vi "Hf Generator - Copy.vi"(4 "Upper Frequency":dbl, 5 "Mic B Comp Fact":dbl, 6 "Speaker Device":dbl, 7 "Mic B":u32, 8 "Duration":dbl) -> (0 "Done":bool, 1 "Outlier Indexes":i32[](array[numeric]), 2 "df":dbl format="%0.2f", 3 "H(f)":cdb[](array[numeric]))   [LabVIEW 2018, in "Impedance Tube.lvlib"]
uses:
  Impedance Tube.lvlib
  <vilib>/sound2/lvsound2.llb/Sound Data Format.ctl
  <vilib>/sound2/lvsound2.llb/Sampling Mode.ctl
  <vilib>/Analysis/4window.llb/windowTd.ctl
  <vilib>/Analysis/6fits.llb/Remove Outliers (Range).vi
  <vilib>/sound2/lvsound2.llb/Sound Input Read (DBL).vi
  <vilib>/measure/maspectr.llb/Frequency Response Function (Real-Im) 1-1.vi
  <vilib>/Analysis/NI_AALPro.lvlib
  <vilib>/measure/NI_MAPro.lvlib
panel:
  out "Waveform Graph 2":dynamicdata(graph)
  out "Waveform Graph":dynamicdata(graph)
  out "Fi":dbl[](graph)
  out "Coherence":cluster{"f0":dbl, "df":dbl, "coherence":dbl[]}(graph)
  out "Numeric":dbl
  out "Frequency  2":cluster{dbl, dbl, dbl[]}(graph)
  out "averages completed":dbl format="%.2p"
  out "initialized array":dbl[](array[numeric])
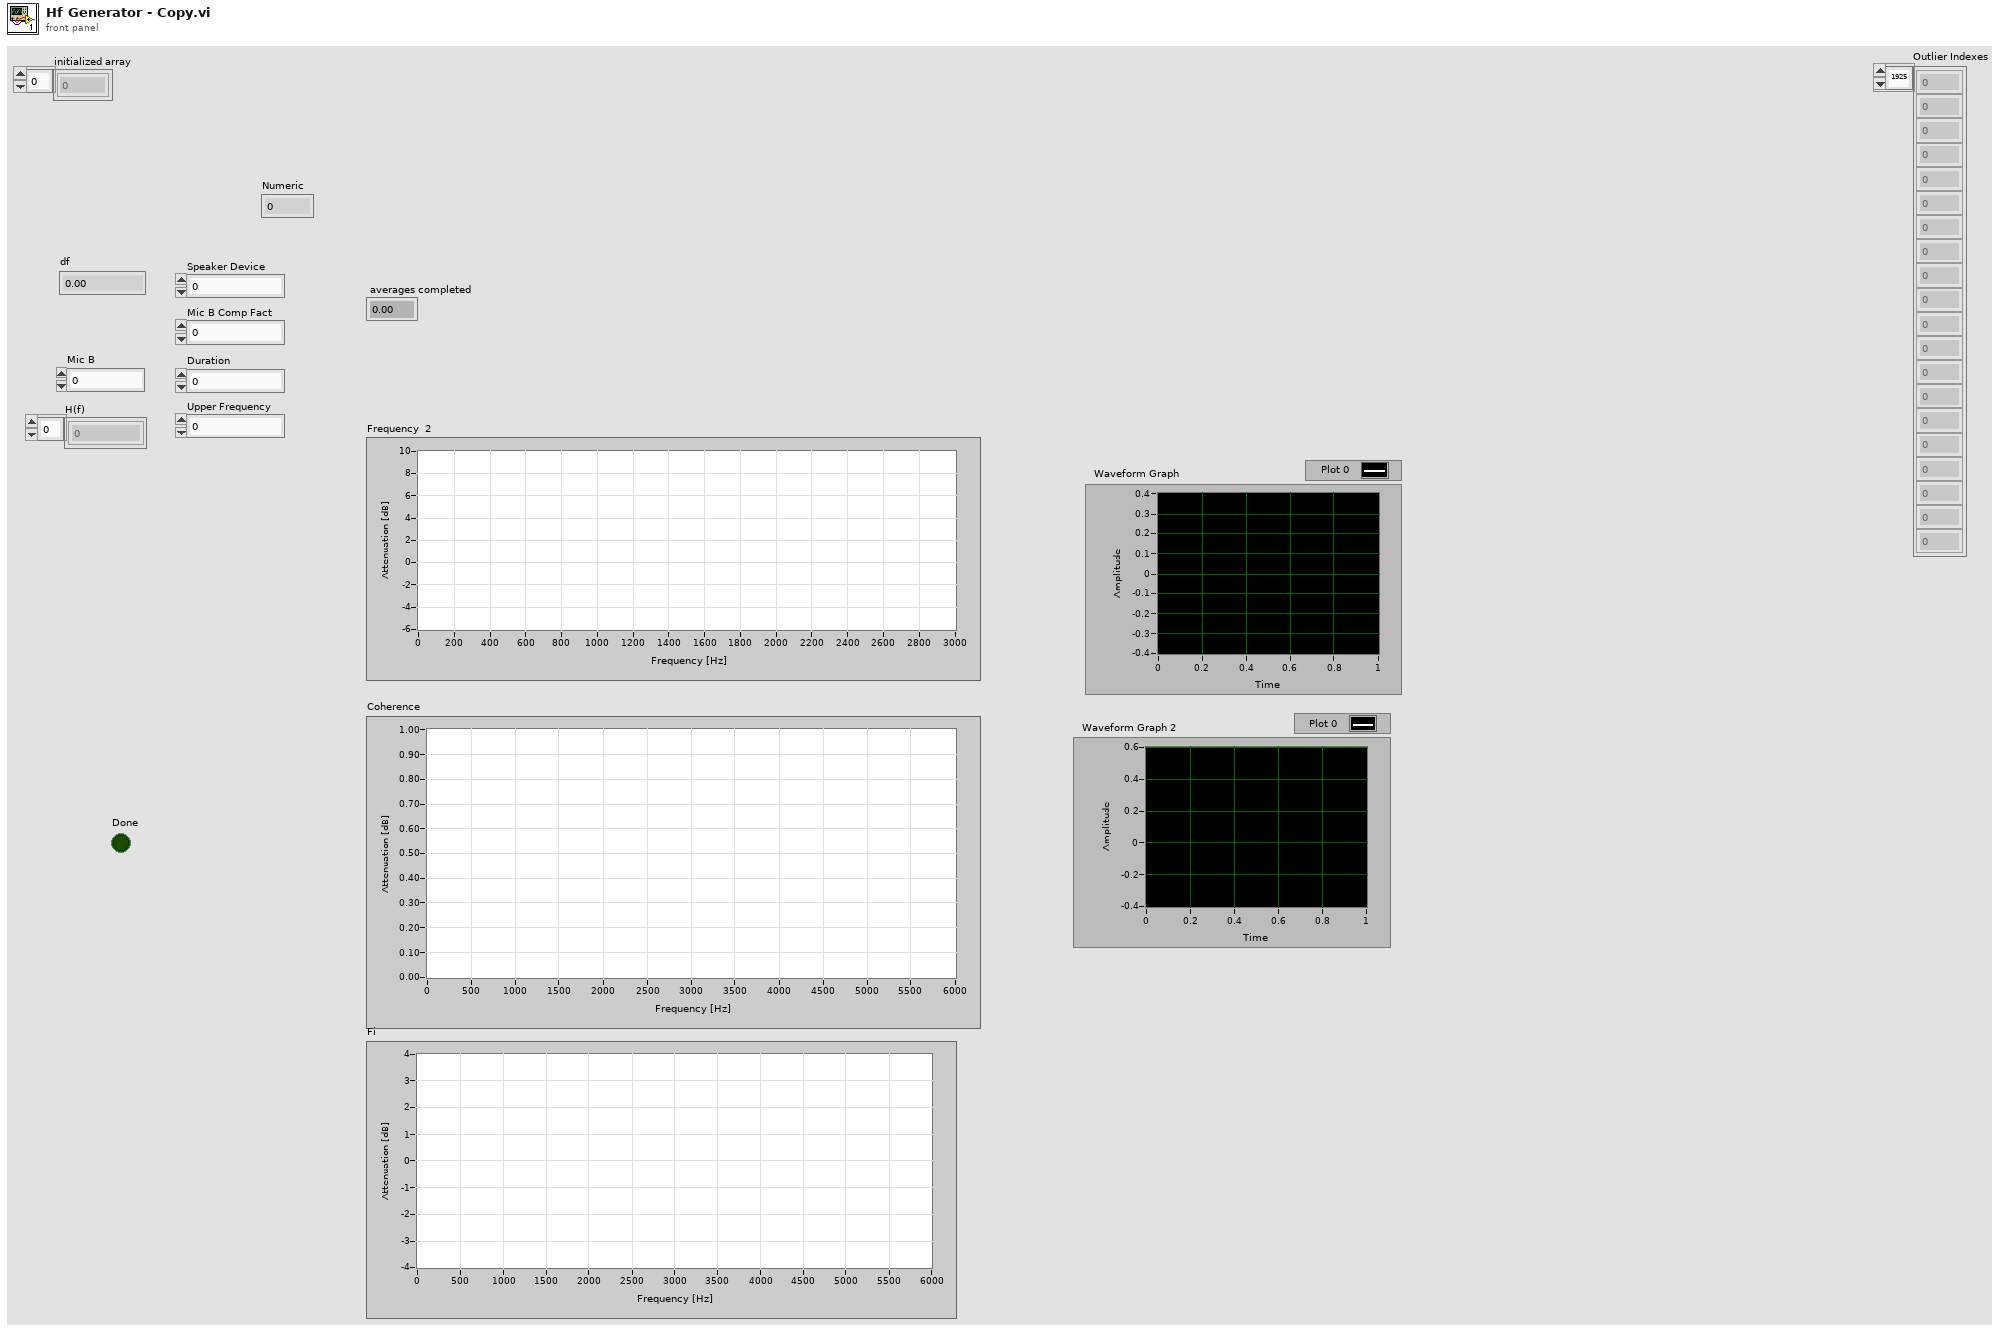
[diagram p1: front panel]
types:
  T1 = cluster{"averaging mode":enum16{"No averaging", "Vector averaging", "RMS averaging", "Peak hold"}, "weighting mode":enum16{"Linear", "Exponential"}, "number of averages":u32}
  T2 = typedef "Sampling Mode.ctl" = i32
  T3 = typedef "Sound Data Format.ctl" = cluster{"sample rate (S/s)":dbl, "number of channels":i32, "bits per sample":i32}
  T4 = typedef "Sound Input Task ID.ctl" = u32
  T5 = typedef "NI_AALPro.lvlib/windowTd.ctl" = u32
  T6 = cluster{"f0":dbl, "df":dbl, "imaginary part":dbl[]}
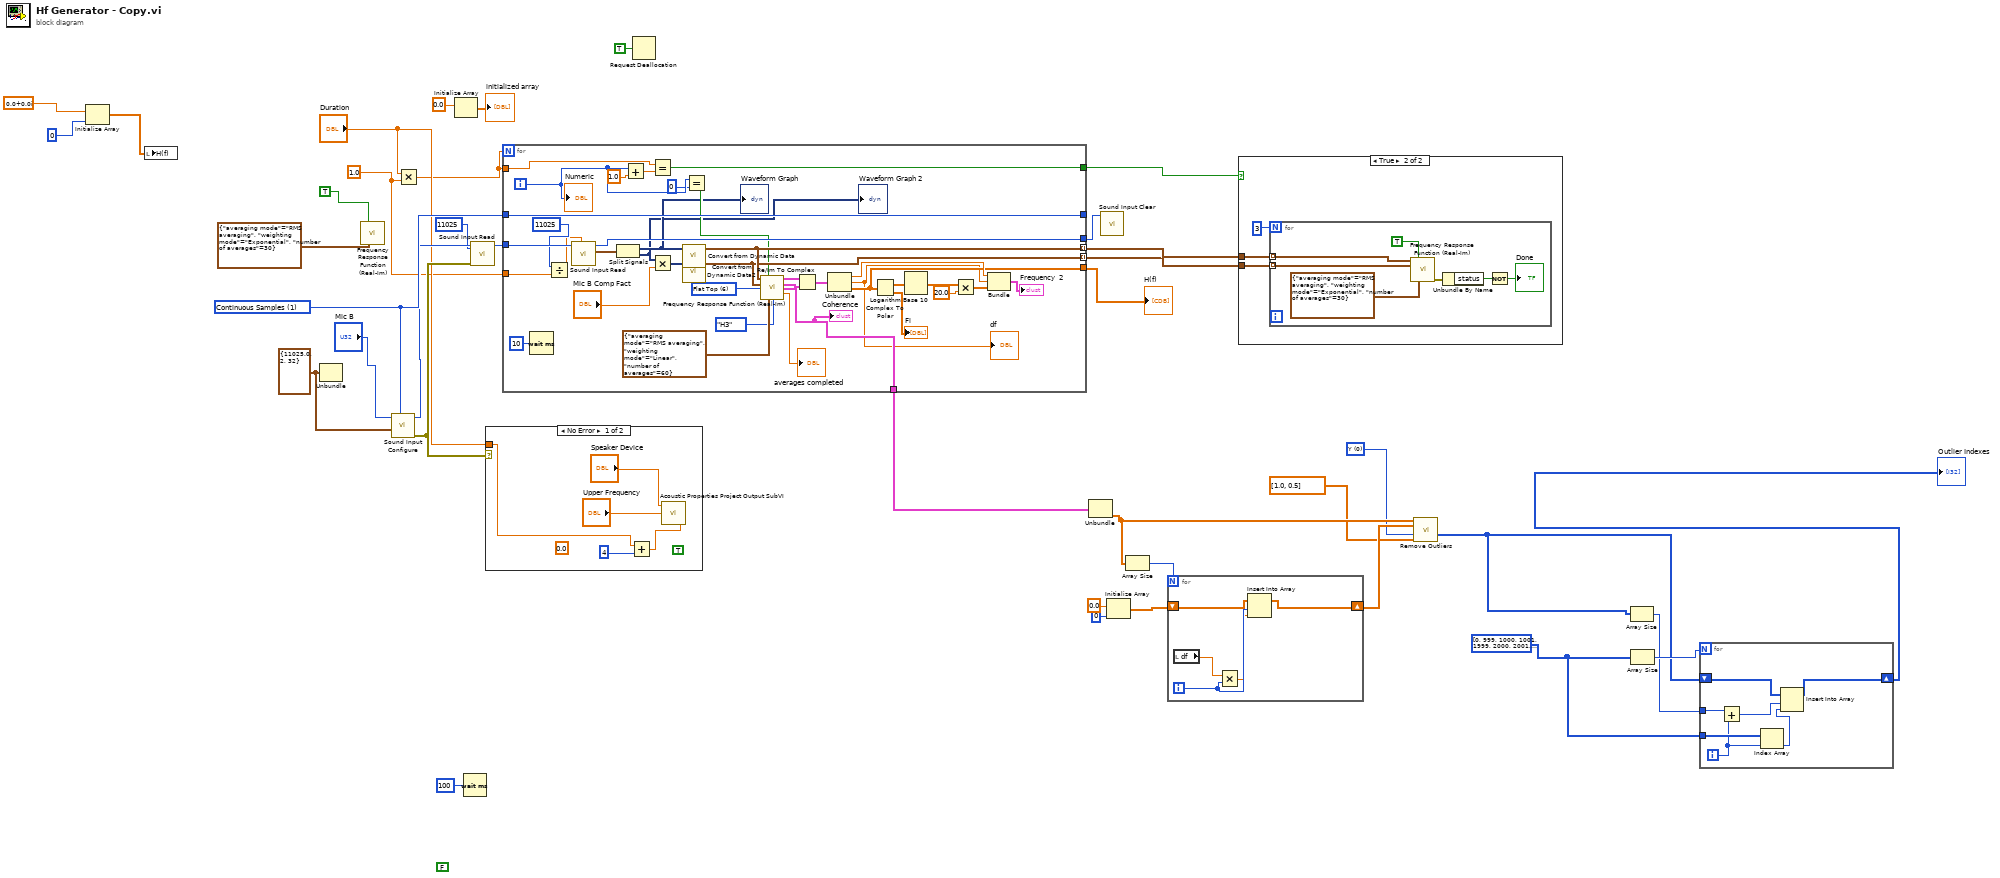
[diagram p0: block diagram]
diagram:
  w5 = i32[] [0, 999, 1000, 1001, 1999, 2000, 2001, 2002] ("element")
  w10 = u16 0 items=["Y", "X", "X and Y"] ("range type")
  w18 = 1.0 ("y")
  w35 = T2 1 items=["Finite Samples", "Continuous Samples"] ("sample mode")
  w36 = T3 {"sample rate (S/s)"=11025.0, "number of channels"=2, "bits per sample"=32} ("sound format")
  (unwired) FALSE
  n1 = Initialize Array(cdb 0.0+0.0i ("element"), 0 ("dimension size")) -> (w1:cdb[])
  n2 = local write "H(f)"(w1) -> ()
  n3 = Unbundle(w36) -> ()  [unwired: 3 out]
  n4 = call-poly <vilib>:"Frequency Response Function (Real-Im).vi"("restart averaging (F)"=TRUE, "averaging parameters"=T1 {"averaging mode"=enum."RMS averaging", "weighting mode"=enum."Exponential", "number of averages"=30}) -> ()  [unwired: 8 in, 6 out]
  n5 = call <vilib>:"Sound Input Configure.vi"("sample mode"=w35, "sound format"=w36, "device ID"="Mic B") -> ("error out"=w22:errorcluster, "task ID"=w31:T4)  [unwired: 7 in]
  n6 = Multiply(x="Duration", y=w18) -> (x*y=w19:dbl)
  n7 = Initialize Array(0.0 ("element")) -> (→"initialized array":dbl[])  [unwired: 1 in]
  n8 = Wait (ms)(milliseconds to wait=u32 100) -> ()  [unwired: 1 out]
  n9 = call-poly <vilib>:"Sound Input Read.vi"("number of samples/ch"=11025, "error in (no error)"=w22, "task ID"=w31) -> ("task ID out"=w30:T4)  [unwired: 6 in, 2 out]
  n10 = case shown="No Error" w22 {
    tunnel: "Duration" -> [w41 _]
    frame No Error {
      (unwired) 0.0 ("Low F")
      (unwired) TRUE ("White Noise")
      n11 = Add(x=w41, y=4) -> (x+y=w39:dbl)
      n12 = call "Acoustic Properties Project Output SubVI.vi"("Duration"=w39, "Upper Frequency"="Upper Frequency", "Speaker Device ID"="Speaker Device") -> ()  [unwired: 2 in]
    }
    frame Error {
    }
  }
  n13 = for {
    N: w19 -> [_]
    tunnel: w30 -> [w81]
    tunnel: w35 -> [w80]
    tunnel: [w79] -> w21
    tunnel: [w80] -> _
    tunnel: w19 -> [w66]
    tunnel: [w51] -> w28
    tunnel: [w60] -> w25 mode=indexing
    tunnel: [w59] -> w24 mode=indexing
    tunnel: [w62] -> w23
    tunnel: w18 -> [w57]
    tunnel: [w49] -> w17
    i -> [w53]
    w76 = T5 6 items=["Rectangle"=0, "Hanning"=1, "Hamming"=2, "Blackman-Harris"=3, "Exact Blackman"=4, "Blackman"=5, "Flat Top"=6, "4 Term B-Harris "=7, "7 Term B-Harris"=8, "Low Sidelobe"=9, "Blackman Nuttall"=11, "Triangle"=30, "Bartlett-Hanning"=31, "Bohman"=32, "Parzen"=33, "Welch"=34, "Kaiser"=60, "Dolph-Chebyshev"=61, "Gaussian"=62] ("window")
    n14 = Wait (ms)(milliseconds to wait=u32 10) -> ()  [unwired: 1 out]
    n15 = Divide(x=11025, y=w57) -> (x/y=w56:dbl)
    n16 = call-poly <vilib>:"Sound Input Read.vi"("number of samples/ch"=w56, "task ID"=w81) -> ("data"=w54:waveform(dbl)[], "task ID out"=w79:T4)  [unwired: 7 in, 1 out]
    n17 = Split Signals(w54) -> (w46:dynamicdata, w45:dynamicdata)  [unwired: 2 in]
    "Waveform Graph" <- w46
    "Waveform Graph 2" <- w45
    n18 = Add(x=w53, y=1.0) -> (x+y=w67:dbl)
    n19 = Equal?(x=w66, y=w67) -> (x = y?=w51:bool)
    n20 = Multiply(x=w45, y="Mic B Comp Fact") -> (x*y=w61:dynamicdata)
    n21 = call "Convert from Dynamic Data"("Dynamic Data Type"=w46) -> ("Waveform"=w60:waveform(dbl))  [unwired: 3 in]
    n22 = call "Convert from Dynamic Data2"("Dynamic Data Type"=w61) -> ("Waveform"=w59:waveform(dbl))  [unwired: 3 in]
    n23 = Equal?(x=w53, y=0) -> (x = y?=w50:bool)
    n24 = call-poly <vilib>:"Frequency Response Function (Real-Im).vi"("time signal X"=w60, "restart averaging (F)"=w50, "time signal Y"=w59, "window"=w76, "averaging parameters"=T1 {"averaging mode"=enum."RMS averaging", "weighting mode"=enum."Linear", "number of averages"=60}, "FRF Mode"=enum16{"H1", "H2", "H3"}."H3") -> ("real part"=w75:cluster{"f0":dbl, "df":dbl, "real part":dbl[]}, "imaginary part"=w74:T6, "coherence"=w49:cluster{"f0":dbl, "df":dbl, "coherence":dbl[]}, "averages completed"=→"averages completed":dbl)  [unwired: 4 in, 2 out]
    "Coherence" <- w49
    n25 = Re/Im To Complex(1:w74, 2:w75) -> (0:w73:cluster{"f0":cdb, "df":cdb, cdb[]})
    n26 = Unbundle(w73) -> ("f0"=w64:cdb, "df"=w48:cdb, w62:cdb[])
    "df" <- w48
    n27 = Complex To Polar(r * e^(i*theta)=w62) -> (r=w70:dbl[], theta=→"Fi":dbl[])
    n28 = Logarithm Base 10(1:w70) -> (0:w72:dbl[])
    n29 = Multiply(x=w72, y=20.0) -> (x*y=w63:dbl[])
    n30 = Bundle("f0"=w64, "df"=w48, w63) -> (→"Frequency  2":cluster{"f0":cdb, "df":cdb, dbl[]})  [unwired: 1 in]
    "Numeric" <- w53
  }
  "H(f)" <- w23
  n31 = Request Deallocation(TRUE ("flag")) -> ()
  n32 = Unbundle(w17) -> ("coherence"=w16:dbl[])  [unwired: 2 out]
  n33 = call <vilib>:"Sound Input Clear.vi"("task ID"=w21) -> ()  [unwired: 10 in, 1 out]
  n34 = Initialize Array(0.0 ("element"), 0 ("dimension size")) -> (w12:dbl[])
  n35 = Array Size(array=w16) -> (size(s)=w15:i32)
  n36 = for {
    N: w15 -> [_]
    shift-right: [w84] -> w11
    shift-left: w12 -> [w85]
    i -> [w83]
    n37 = local read "df"() -> (w86:dbl)
    n38 = Multiply(x=w86, y=w83) -> (x*y=w82:dbl)
    n39 = Insert Into Array(array=w85, index=w83, new element=w82) -> (w84:dbl[])
  }
  n40 = case shown="True" w28 {
    tunnel: w25 -> [_ w89]
    tunnel: w24 -> [_ w88]
    frame False {
    }
    frame True {
      n41 = for {
        N: 3 -> [_]
        tunnel: w89 -> [w91] mode=indexing
        tunnel: w88 -> [w90] mode=indexing
        n42 = call-poly <vilib>:"Frequency Response Function (Real-Im).vi"("time signal X"=w91, "restart averaging (F)"=TRUE, "time signal Y"=w90, "averaging parameters"=T1 {"averaging mode"=enum."RMS averaging", "weighting mode"=enum."Exponential", "number of averages"=30}) -> ("error out"=w93:errorcluster)  [unwired: 6 in, 5 out]
        n43 = Unbundle By Name(w93) -> ("status"=w94:bool)
        n44 = Not(x=w94) -> (.not. x?=→"Done":bool)
      }
    }
  }
  n45 = call-poly <vilib>:"Remove Outliers.vi"("Y"=w16, "X"=w11, "range type"=w10, "Range"=dbl[] [1.0, 0.5]) -> ("Outlier Indexes"=w7:i32[])  [unwired: 7 in, 4 out]
  n46 = Array Size(array=w7) -> (size(s)=w6:i32)
  n47 = Array Size(array=w5) -> (size(s)=w8:i32)
  n48 = for {
    N: w8 -> [_]
    shift-right: [w102] -> w4
    shift-left: w7 -> [w103]
    tunnel: w6 -> [w101]
    tunnel: w5 -> [w99]
    i -> [w98]
    n49 = Add(x=w101, y=w98) -> (x+y=w100:i32)
    n50 = Index Array(array=w99, index=w98) -> (element=w97:i32)
    n51 = Insert Into Array(array=w103, index=w100, new element=w97) -> (w102:i32[])
  }
  "Outlier Indexes" <- w4
